vi "Lockin.DAQ.Create.vi"(8 "error in":errorcluster, 11 "Lockin.DAQ":refnum<class "Lockin.DAQ.lvclass">) -> (0 "error out":errorcluster, 3 "Lockin.DAQ":refnum<class "Lockin.DAQ.lvclass">)   [LabVIEW 2016, in "Lockin.DAQ.lvclass"]
uses:
  Lockin.DAQ.lvclass
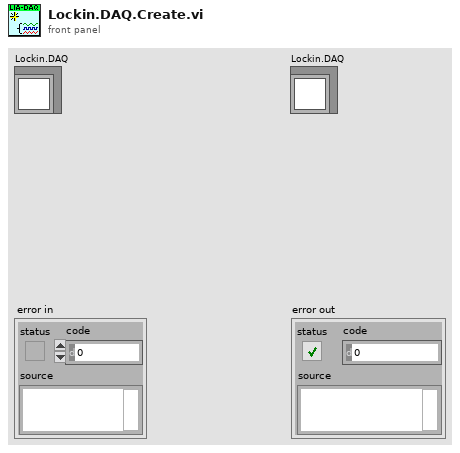
[diagram p1: front panel]
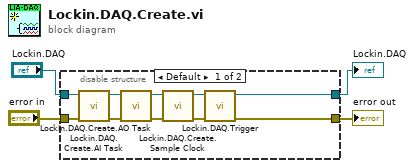
[diagram p0: block diagram]
diagram:
  n1 = disable-structure shown="Default" {
    disable-tunnel: "Lockin.DAQ" -> [w8 w16]
    disable-tunnel: "error in" -> [w7 w15]
    disable-tunnel: [w6 w16] -> w2
    disable-tunnel: [w5 w15] -> w1
    frame condition #0 (active) {
      n2 = call "Lockin.DAQ.Create.AI Task.vi"("error in (no error)"=w7, "Lockin.DAQ"=w8) -> ("error out"=w9:errorcluster, "Lockin.DAQ"=w10:refnum<class "Lockin.DAQ.lvclass">)  [unwired: 8 in]
      n3 = call "Lockin.DAQ.Create.AO Task.vi"("error in (no error)"=w9, "Lockin.DAQ"=w10) -> ("error out"=w11:errorcluster, "Lockin.DAQ"=w12:refnum<class "Lockin.DAQ.lvclass">)  [unwired: 8 in]
      n4 = call "Lockin.DAQ.Create.Sample Clock.vi"("error in (no error)"=w11, "Lockin.DAQ"=w12) -> ("error out"=w13:errorcluster, "Lockin.DAQ"=w14:refnum<class "Lockin.DAQ.lvclass">)  [unwired: 8 in]
      n5 = call "Lockin.DAQ.Trigger.vi"("error in (no error)"=w13, "Lockin.DAQ"=w14) -> ("error out"=w5:errorcluster, "Lockin.DAQ"=w6:refnum<class "Lockin.DAQ.lvclass">)  [unwired: 8 in]
    }
    frame condition #1 {
    }
  }
  "error out" <- w1
  "Lockin.DAQ" <- w2
